vi "通讯全局变量.vi"() -> ()   [LabVIEW 2016, in "环境动力监测库.lvlib" / "浮标电源管理.lvlib"]
uses:
  <vilib>/Plasmionique/MB Master/MB_Master/MB_Master.lvclass
panel:
  in  "MPPT":T1
  in  "参数":T2={"低压报警阈值 V"=21.0, "低压报警解除阈值 V"=21.0, "高温报警阈值 ℃"=50.0, "高温报警解除阈值 ℃"=50.0, "湿度报警阈值 %"=95.0, "湿度报警解除阈值 %"=95.0}
  out "输出簇":T3
  out "MB session":refnum<class "MB_Master.lvclass">
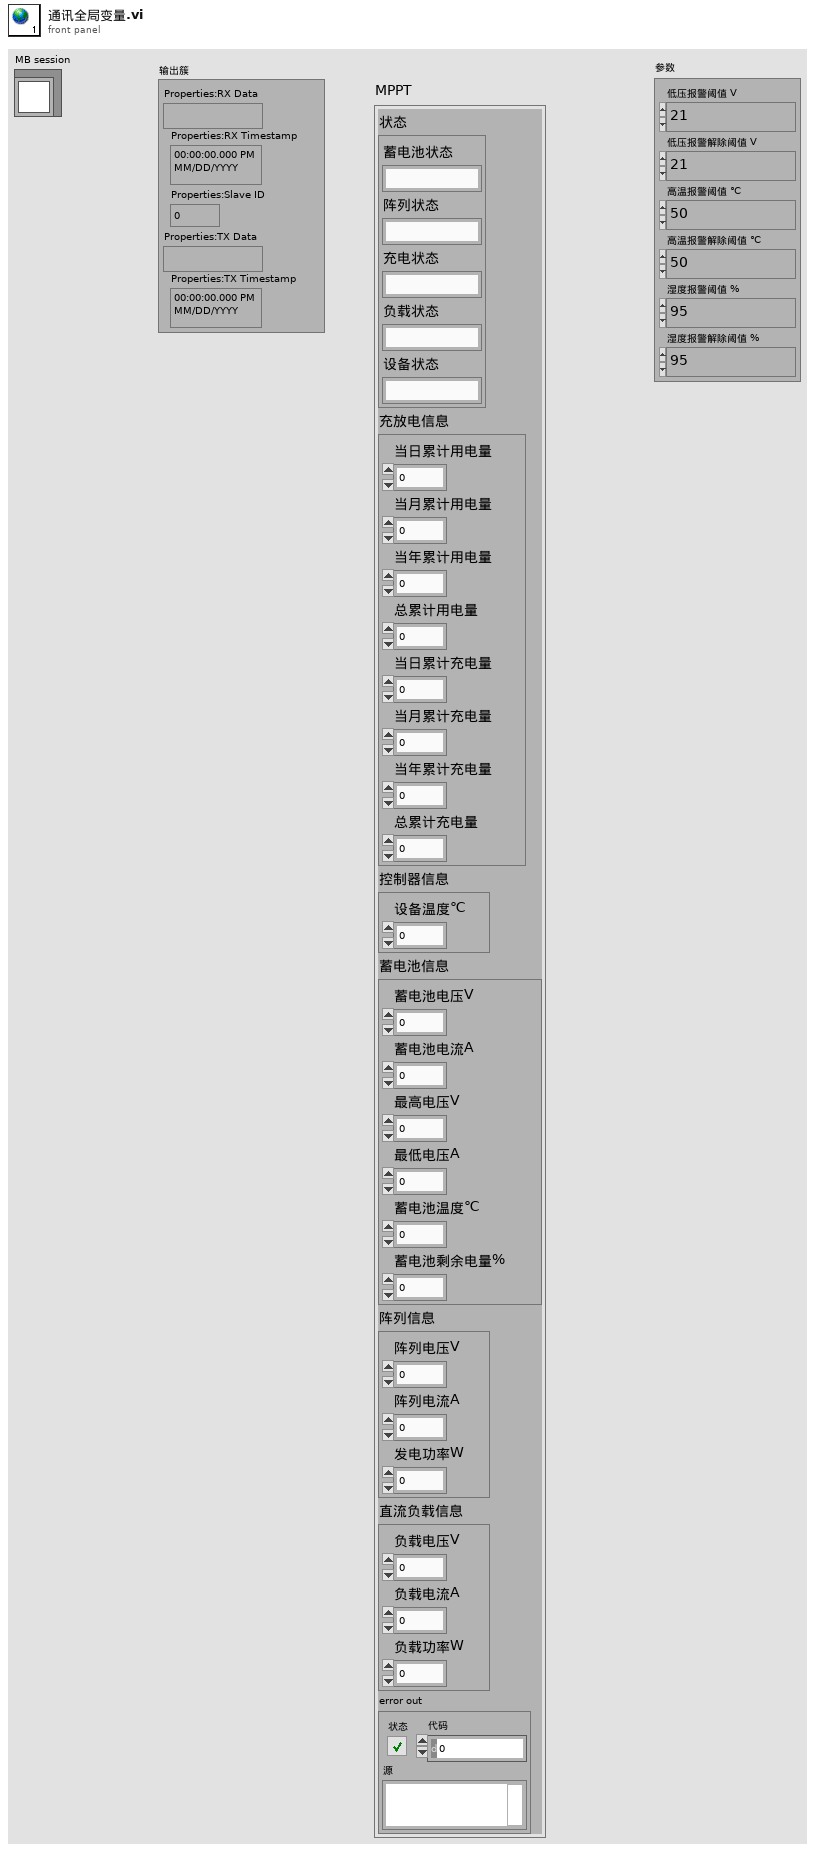
[diagram p1: front panel]
types:
  T1 = cluster{"状态":cluster{"蓄电池状态":string, "阵列状态":string, "充电状态":string, "负载状态":string, "设备状态":string}, "充放电信息":cluster{"当日累计用电量":sgl, "当月累计用电量":sgl, "当年累计用电量":sgl, "总累计用电量":sgl, "当日累计充电量":sgl, "当月累计充电量":sgl, "当年累计充电量":sgl, "总累计充电量":sgl}, "控制器信息":cluster{"设备温度℃":dbl}, "蓄电池信息":cluster{"蓄电池电压V":dbl, "蓄电池电流A":dbl, "最高电压V":dbl, "最低电压A":dbl, "蓄电池温度℃":dbl, "蓄电池剩余电量%":dbl}, "阵列信息":cluster{"阵列电压V":dbl, "阵列电流A":dbl, "发电功率W":dbl}, "直流负载信息":cluster{"负载电压V":dbl, "负载电流A":dbl, "负载功率W":dbl}, "error out":errorcluster}
  T2 = cluster{"低压报警阈值 V":dbl, "低压报警解除阈值 V":dbl, "高温报警阈值 ℃":dbl, "高温报警解除阈值 ℃":dbl, "湿度报警阈值 %":dbl, "湿度报警解除阈值 %":dbl}
  T3 = cluster{"Properties:RX Data":string, "Properties:RX Timestamp":timestamp, "Properties:Slave ID":u8, "Properties:TX Data":string, "Properties:TX Timestamp":timestamp}
diagram:
